vi "PID Lead.vi"(7 "Set? (F:Read)":bool, 8 "Error In":errorcluster, 9 "Lead (0)":dbl[unit], 11 "VISA resource name":refnum<visa-resource-name>) -> (0 "Error Out":errorcluster, 1 "Lead out":dbl[unit], 3 "dup VISA resource name":refnum<visa-resource-name>)   [LabVIEW 2016, in "MGC647C.lvlib"]
doc: "Read/Set PID lead parameter."
uses:
  MGC647C.lvlib
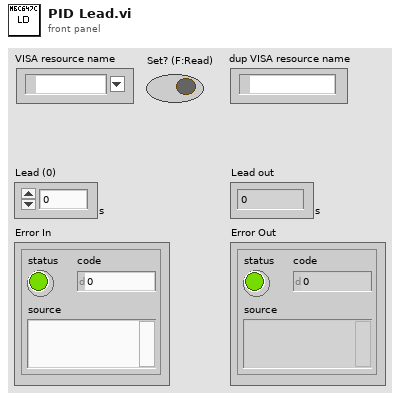
[diagram p1: front panel]
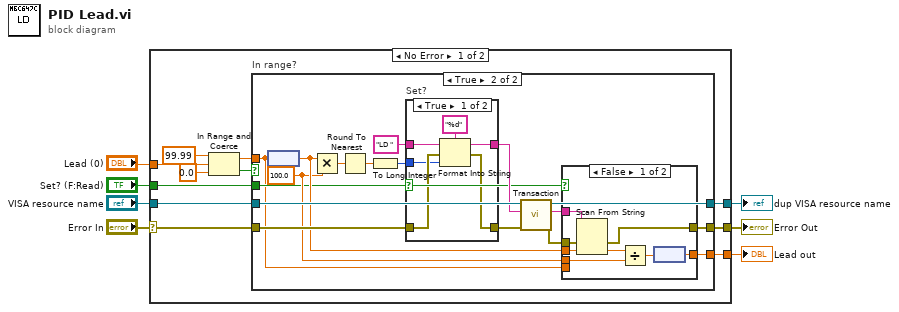
[diagram p0: block diagram]
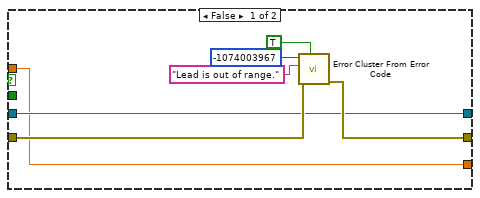
[diagram p2: hidden frame]
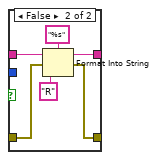
[diagram p4: hidden frame]
diagram:
  n1 = case shown="No Error" "Error In" {
    selector: "Error In" -> [w10 w66]
    tunnel: "VISA resource name" -> [w18 w65]
    tunnel: [w17 w65] -> w6
    tunnel: [w16 w66] -> w5
    tunnel: "Set? (F:Read)" -> [w15 _]
    tunnel: "Lead (0)" -> [w14 w67]
    tunnel: [w9 w67] -> w1
    frame No Error {
      n2 = In Range and Coerce(upper limit=dbl[unit] 99.99, x=w14, lower limit=dbl[unit] 0.0) -> (coerced(x)=w13:dbl[unit], In Range?=w8:bool)
      n3 = case "In range?" shown="True" w8 {
        tunnel: w18 -> [w23 w42]
        tunnel: [w23 w41] -> w17
        tunnel: [w24 w36] -> w16
        tunnel: w15 -> [_ w27]
        tunnel: w13 -> [w22 w26]
        tunnel: w10 -> [w25 w40]
        tunnel: [w22 w28] -> w9
        frame False {
          n4 = call <vilib>:"Error Cluster From Error Code.vi"("show call chain? (False)"=TRUE, "error in (no error)"=w25, "error message (\"\")"="Lead is out of range." ("error message (\"\")"), "error code (0)"=-1074003967) -> ("error out"=w24:errorcluster)  [unwired: 5 in]
        }
        frame True {
          w29 = 100.0 ("x")
          n5 = node(w26) -> (w33:dbl)
          n6 = Multiply(x=w33, y=w29) -> (x*y=w32:dbl)
          n7 = Round To Nearest(number=w32) -> (nearest integer value=w31:dbl)
          n8 = To Long Integer(number=w31) -> (32bit integer=w30:i32)
          n9 = case "Set?" shown="True" w27 {
            tunnel: w40 -> [w58 w64]
            tunnel: [w57 w63] -> w39
            tunnel: w30 -> [w56 _]
            tunnel: "LD " ("string (\"\")") -> [w55 w62]
            tunnel: [w54 w61] -> w34
            frame True {
              n10 = Format Into String(format string="%d", initial string=w55, error in=w58, w56) -> (resulting string=w54:string, error out=w57:errorcluster)
            }
            frame False {
              n11 = Format Into String(format string="%s", initial string=w62, error in=w64, "R") -> (resulting string=w61:string, error out=w63:errorcluster)
            }
          }
          n12 = call "Transaction.vi"("Error In"=w39, "Command"=w34, "VISA resource name"=w42) -> ("Error Out"=w37:errorcluster, "Response"=w38:string, "dup VISA resource name"=w41:refnum<visa-resource-name>)  [unwired: 6 in]
          n13 = case shown="False" w27 {
            tunnel: w38 -> [w50 _]
            tunnel: w37 -> [w49 w52]
            tunnel: [w48 w52] -> w36
            tunnel: w33 -> [w47 _]
            tunnel: w29 -> [w45 _]
            tunnel: [w43 w51] -> w28
            tunnel: w26 -> [_ w51]
            frame False {
              n14 = Scan From String(input string=w50, error in=w49, default 1=w47) -> (error out=w48:errorcluster, output 1=w46:dbl)  [unwired: 2 in, 2 out]
              n15 = Divide(x=w46, y=w45) -> (x/y=w44:dbl)
              n16 = node(w44) -> (w43:dbl[unit])
            }
            frame True {
            }
          }
        }
      }
    }
    frame Error {
    }
  }
  "dup VISA resource name" <- w6
  "Error Out" <- w5
  "Lead out" <- w1
